vi "VI Tree.vi"   [LabVIEW 2015, in "Fluke 289.lvlib"]
doc: "This is the instrument driver for the Fluke 287 and Fluke 289. The VI Tree displays all the user-callable VIs of the instrument driver in an organized table."
uses:
  <instrlib>/Fluke 289/Fluke 289.lvlib
panel:
  # "(c) 2014 National Instruments.  ALL RIGHTS RESERVED."
  # "SEE DIAGRAM\nFOR VI TREE."
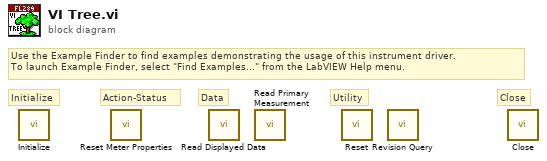
[diagram p0: block diagram]
diagram:
  # "Close"
  # "Utility"
  # "Data"
  # "Action-Status"
  # "Initialize"
  # "Use the Example Finder to find examples demonstrating the usage of this instrument driver.\nTo launch Example Finder, select \"Find Examples...\" from the LabVIEW Help menu."
  n1 = call <instrlib>:"Initialize.vi"() -> ()  [unwired: 10 in, 2 out]
  n2 = call <instrlib>:"Reset Meter Properties.vi"() -> ()  [unwired: 10 in, 2 out]
  n3 = call <instrlib>:"Read Displayed Data.vi"() -> ()  [unwired: 9 in, 3 out]
  n4 = call <instrlib>:"Read Primary Measurement.vi"() -> ()  [unwired: 6 in, 6 out]
  n5 = call <instrlib>:"Reset.vi"() -> ()  [unwired: 10 in, 2 out]
  n6 = call <instrlib>:"Revision Query.vi"() -> ()  [unwired: 8 in, 4 out]
  n7 = call <instrlib>:"Close.vi"() -> ()  [unwired: 11 in, 1 out]
